vi "dfd_Lattice AR to TF.vi"(9 "gain":dbl=1.0 format="%.2f", 10 "k [1~M]":dbl[](array[numeric]) format="%.2f") -> (2 "denominator":dbl[](array[numeric]) format="%.2f", 3 "numerator":dbl[](array[numeric]))   [LabVIEW 2017, in "NI_DigFilterLicensed.lvlib"]
uses:
  <vilib>/addons/Digital Filter Design/NI_DigFilterLicensed.lvlib
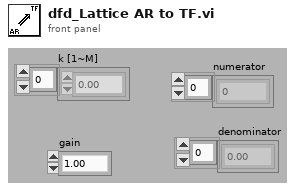
[diagram p1: front panel]
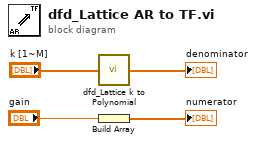
[diagram p0: block diagram]
diagram:
  n1 = call <vilib>:"dfd_Lattice k to Polynomial.vi"("k"="k [1~M]") -> ("poly"=→"denominator":dbl[])
  n2 = Build Array("gain") -> (→"numerator":dbl[])
